vi "clone.vi"(0 "reference":refnum<class "ClassNode.lvclass">, 5 "error in (no error)":errorcluster) -> (14 "reference out":refnum<class "ClassNode.lvclass">, 15 "clonedClassNode":refnum<class "AbstractNode.lvclass">, 19 "error out":errorcluster)   [LabVIEW 2012, in "ClassNode.lvclass"]
doc: "public Object clone()"
uses:
  <resource>/Framework/Providers/Open_GDS/UML/ClassNode_class/ClassNode.lvclass
  <resource>/Framework/Providers/Open_GDS/UML/AbstractNode_class/AbstractNode.lvclass
  <resource>/Framework/Providers/Open_GDS/UML/MultiLineString_class/MultiLineString.lvclass
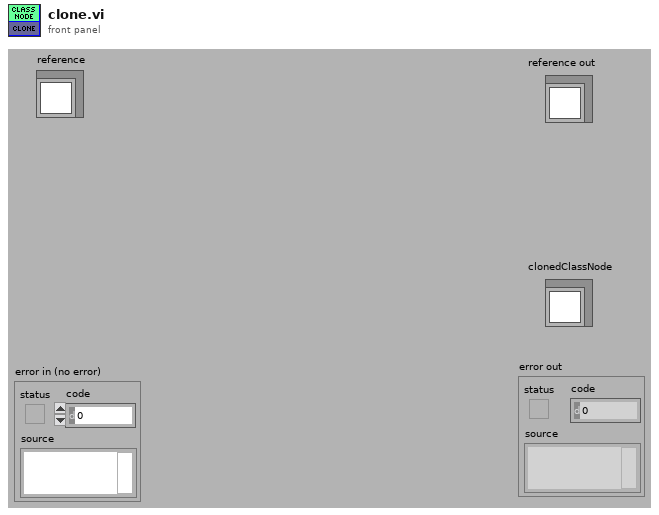
[diagram p1: front panel]
types:
  T1 = typedef "ClassNode.lvclass/ObjectAttributes.ctl" = cluster{"Base class":T2, "midHeight":dbl, "botHeight":dbl, "name":refnum<class "MultiLineString.lvclass">, "attributes":refnum<class "MultiLineString.lvclass">, "methods":refnum<class "MultiLineString.lvclass">, "DEFAULT_COMPARTMENT_HEIGHT":i32, "DEFAULT_WIDTH":i32, "DEFAULT_HEIGHT":i32, "showMethods":bool, "showAttributes":bool, "ClassPath":path}
  T2 = typedef "RectangularNode.lvclass/ObjectAttributes.ctl" = cluster{"Base class":T3, "bounds":T4}
  T3 = typedef "AbstractNode.lvclass/ObjectAttributes.ctl" = cluster{"parent":refnum<class "AbstractNode.lvclass">, "children":refnum<class "AbstractNode.lvclass">[], "Hidden":bool}
  T4 = typedef "Rectangle Rectangle2D.ctl" = cluster{"x":dbl, "y":dbl, "width":dbl, "height":dbl}
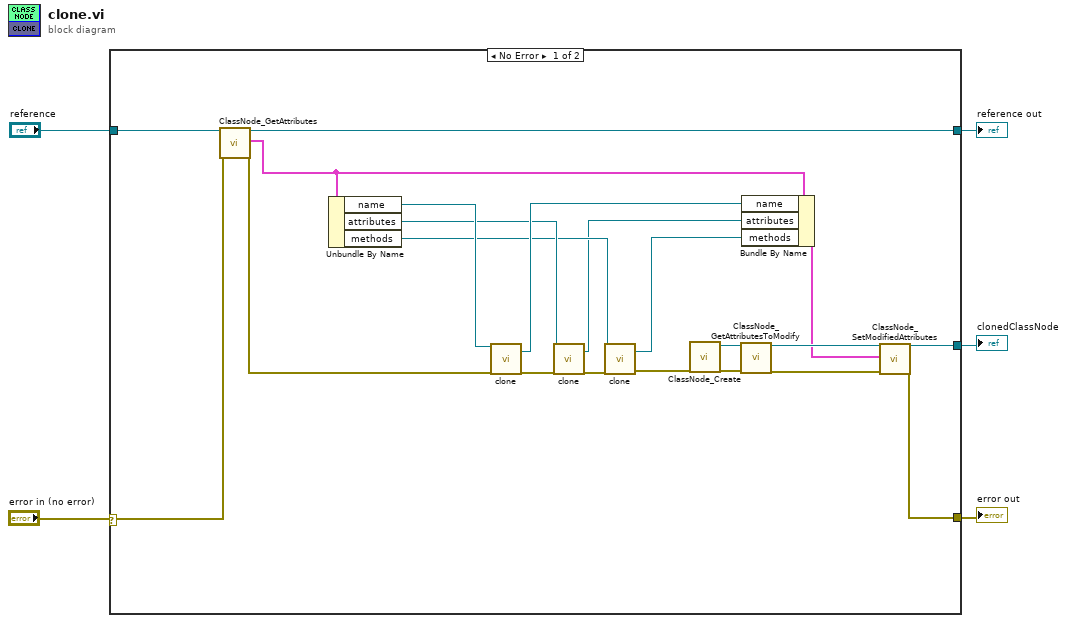
[diagram p0: block diagram]
diagram:
  n1 = case shown="No Error" "error in (no error)" {
    selector: "error in (no error)" -> [w24 w27]
    tunnel: "reference" -> [w26 w28]
    tunnel: [w25 w27] -> w4
    tunnel: [w6 w28] -> w3
    tunnel: [w23 _] -> w1
    frame No Error {
      n2 = call <resource>:"ClassNode_GetAttributes.vi"("reference in"=w26, "error in (no error)"=w24) -> ("reference out"=w6:refnum<class "ClassNode.lvclass">, "Attributes"=w11:T1, "error out"=w10:errorcluster)  [unwired: 15 out]
      n3 = Unbundle By Name(w11) -> ("name"=w19:refnum<class "MultiLineString.lvclass">, "attributes"=w15:refnum<class "MultiLineString.lvclass">, "methods"=w14:refnum<class "MultiLineString.lvclass">)
      n4 = call-dynamic "clone.vi"("reference"=w19, "error in (no error)"=w10) -> ("clonedMultiLineString"=w18:refnum<class "MultiLineString.lvclass">, "error out"=w17:errorcluster)  [unwired: 15 in, 1 out]
      n5 = call-dynamic "clone.vi"("reference"=w15, "error in (no error)"=w17) -> ("clonedMultiLineString"=w13:refnum<class "MultiLineString.lvclass">, "error out"=w16:errorcluster)  [unwired: 15 in, 1 out]
      n6 = call-dynamic "clone.vi"("reference"=w14, "error in (no error)"=w16) -> ("clonedMultiLineString"=w12:refnum<class "MultiLineString.lvclass">, "error out"=w7:errorcluster)  [unwired: 15 in, 1 out]
      n7 = call <resource>:"ClassNode_Create.vi"("error in (no error)"=w7) -> ("reference out"=w9:refnum<class "ClassNode.lvclass">, "error out"=w8:errorcluster)  [unwired: 16 in, 1 out]
      n8 = call <resource>:"ClassNode_GetAttributesToModify.vi"("reference in"=w9, "error in (no error)"=w8) -> ("reference out"=w22:refnum<class "ClassNode.lvclass">, "error out"=w21:errorcluster)  [unwired: 1 in, 15 out]
      n9 = Bundle By Name(cluster=w11, "name"=w18, "attributes"=w13, "methods"=w12) -> (w20:T1)
      n10 = call <resource>:"ClassNode_SetModifiedAttributes.vi"("reference in"=w22, "Attributes"=w20, "error in (no error)"=w21) -> ("reference out"=w23:refnum<class "ClassNode.lvclass">, "error out"=w25:errorcluster)  [unwired: 3 in, 12 out]
    }
    frame Error {
    }
  }
  "reference out" <- w3
  "error out" <- w4
  "clonedClassNode" <- w1
